vi "Pre Launch Init.vi"(11 "WebSocket Client in":refnum<class "WebSocket Client.lvclass">) -> (0 "error out":errorcluster, 3 "WebSocket Client out":refnum<class "WebSocket Client.lvclass">)   [LabVIEW 2016, in "WebSocket Actors.lvlib" / "WebSocket Client.lvclass"]
doc: "(<B>Filename</B>: Actor Framework.lvlib:Actor.lvclass:Pre Launch Init.vi)\n\nDefines behavior that occurs after the Launch Nested Actor method is invoked but before the actor's Actor Core method begins running.\n\nBy default, this method does nothing. A descendant class may override it to define behavior."
uses:
  WebSocket Client.lvclass
  C:/Projects/Shared Libraries/WebSocket Actor/WebSocket Actor/WebSocket Connection/WebSocket Connection.lvclass
  WebSocket Client.lvclass/WebSocket Client.ctl
  WebSocket Connection/WebSocket Connection.lvclass/WebSocket Connection.ctl
  WebSocket Connection/properties/Write WebSocket Connection.vi
  WebSocket Connection/properties/Write Peer ID.vi
  WebSocket Connection/WebSocket Connection.lvclass
  WebSockets/WebSockets.lvlib
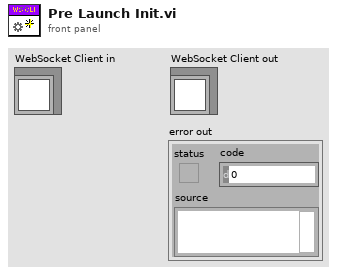
[diagram p1: front panel]
types:
  T1 = typedef "WebSockets.lvlib/Headers.ctl" = cluster{"Name":string, "Value":string}
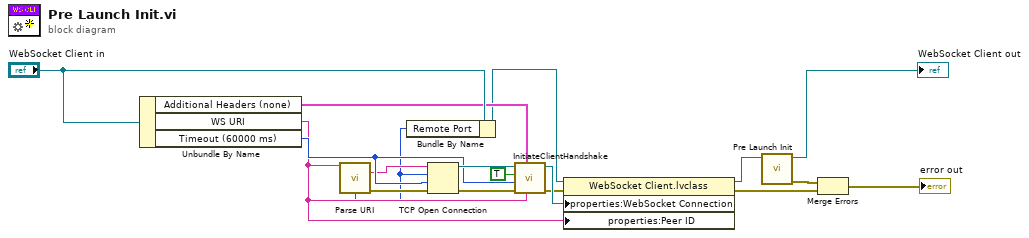
[diagram p0: block diagram]
diagram:
  n1 = Unbundle By Name("WebSocket Client in") -> ("Additional Headers (none)"=w15:T1[], "WS URI"=w6:string, "Timeout (60000 ms)"=w12:i32)
  n2 = call "Parse URI.vi"("URI"=w6) -> ("Hostname"=w3:string, "Port"=w1:u16, "error out"=w5:errorcluster)  [unwired: 8 in, 4 out]
  n3 = Bundle By Name(cluster="WebSocket Client in", "Remote Port"=w1) -> (w4:refnum<class "WebSocket Client.lvclass">)
  n4 = TCP Open Connection(address=w3, remote port or service name=w1, timeout ms (60000)=w12, error in (no error)=w5) -> (connection ID=w14:refnum<k5>, error out=w13:errorcluster)  [unwired: 1 in]
  n5 = call "InitiateClientHandshake.vi"("WS URI"=w6, "additional headers (none)"=w15, "error in (no error)"=w13, "timeout ms (5000)"=w12, "Relative URI Request (F)"=TRUE, "WebSocket Connection in"=w14) -> ("error out"=w9:errorcluster, "WebSocket Connection out"=w10:refnum<k5>)  [unwired: 3 in, 1 out]
  n6 = property class="WebSocket Client.lvclass"(reference=w4, error in=w9, "properties:WebSocket Connection"=w10, "properties:Peer ID"=w6) -> (reference out=w11:refnum<class "WebSocket Client.lvclass">, error out=w7:errorcluster)
  n7 = call-parent "Pre Launch Init.vi"("Monitored Actor in"=w11) -> ("error out"=w18:errorcluster, "Monitored Actor out"=→"WebSocket Client out":refnum<class "WebSocket Client.lvclass">)  [unwired: 9 in]
  n8 = Merge Errors(w18, w7) -> (→"error out":errorcluster)
